vi "Read_configFile_for_Target.vi"(1 "error in":errorcluster, 6 "Target File Path":path, 7 "Ring 2":u16(ring) items=["Target Nmae", "OS Flavour", "Filter  Rates", "Avoid Rates"], 8 "Target Name":string) -> (0 "error out":errorcluster, 2 "selected target":string)   [LabVIEW 2015]
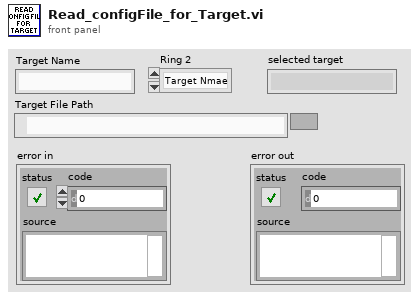
[diagram p1: front panel]
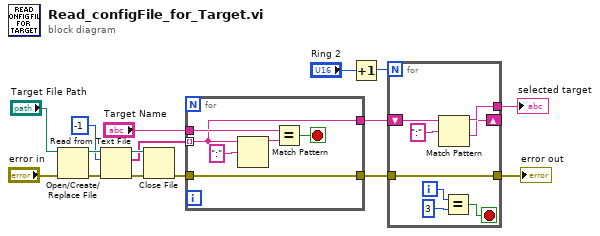
[diagram p0: block diagram]
diagram:
  n1 = Open/Create/Replace File(file path (use dialog)="Target File Path", error in="error in") -> (refnum out=w16:refnum<file>, error out=w15:errorcluster)  [unwired: 4 in, 1 out]
  n2 = Read from Text File(file (use dialog)=w16, count=-1, error in=w15) -> (refnum out=w13:refnum<file>, text=w11:string[], error out=w14:errorcluster)  [unwired: 1 in, 1 out]
  n3 = Close File(refnum=w13, error in=w14) -> (error out=w4:errorcluster)  [unwired: 1 out]
  n4 = for {
    tunnel: w11 -> [w18] mode=indexing
    tunnel: "Target Name" -> [w20]
    tunnel: [w18] -> w7
    tunnel: w4 -> [w17]
    tunnel: [w17] -> w3
    stop <- w19 stop-if-true
    n5 = Match Pattern(string=w18, regular expression=":") -> (before substring=w21:string)  [unwired: 1 in, 3 out]
    n6 = Equal?(x=w20, y=w21) -> (x = y?=w19:bool)
  }
  n7 = Increment(x="Ring 2") -> (x+1=w8:u16)
  n8 = for {
    N: w8 -> [_]
    shift-right: [w24] -> _
    shift-left: w7 -> [w26]
    tunnel: [w25] -> w6
    tunnel: w3 -> [w23]
    tunnel: [w23] -> w2
    i -> [w27]
    stop <- w28 stop-if-true
    n9 = Match Pattern(string=w26, regular expression=":") -> (before substring=w25:string, after substring=w24:string)  [unwired: 1 in, 2 out]
    n10 = Equal?(x=w27, y=3) -> (x = y?=w28:bool)
  }
  "selected target" <- w6
  "error out" <- w2
